vi "Impedance tube v1.0.1.vi"() -> ()   [LabVIEW 2021]
uses:
  <vilib>/Analysis/1siggen.llb/Ramp Pattern by Samples.vi
  <vilib>/express/express analysis/Spectral/Block/exnSpectralBlock spectral measurements RMS poly.vi
  <vilib>/express/express analysis/Spectral/Block/exnSpectralBlock spectral measurements RMS DDT.vi
  <vilib>/express/express arith-compare/Formula/XNode/ExpressFormulaBlockNode.xnode
  <vilib>/express/express analysis/Spectral/XNode/ExpressSpectralMeasurementsBlockNode.xnode
  <vilib>/Analysis/NI_AALPro.lvlib
  <vilib>/Analysis/NI_AALBase.lvlib
panel:
  out "Probe":dbl[](graph)
  out "Rr":dbl[](graph)
  out "Absorption coeff":dbl[](graph)
  in  "number of samples":i32=2048
  out "MIC 2":dynamicdata(graph)
  out "MIC 2":dbl
  out "FFT1":dynamicdata(graph)
  out "MIC 1":dynamicdata(graph)
  out "MIC 1":dbl
  in  "stop (F)":bool
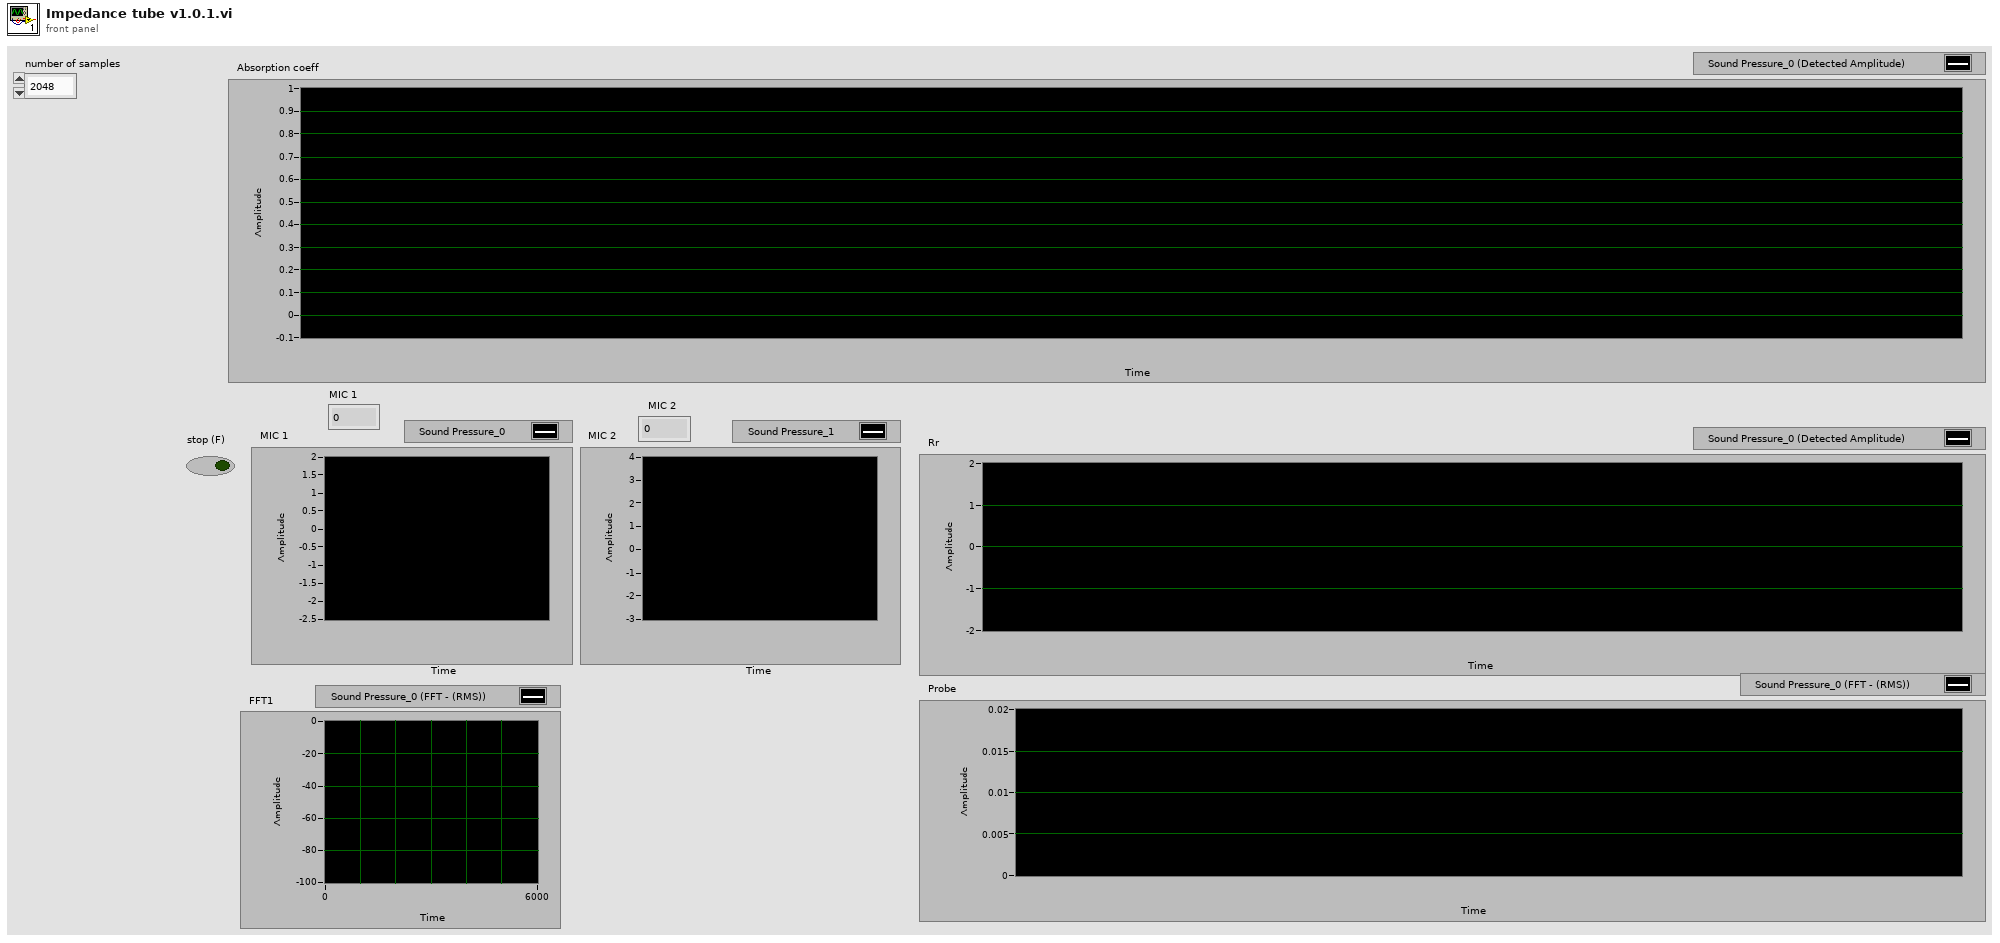
[diagram p1: front panel]
types:
  T1 = cluster{"averaging mode":u16, "weighting mode":u16, "number of averages":u32}
  T2 = cluster{"dB On (F)":bool, "unwrap phase (F)":bool, "convert to degree (F)":bool}
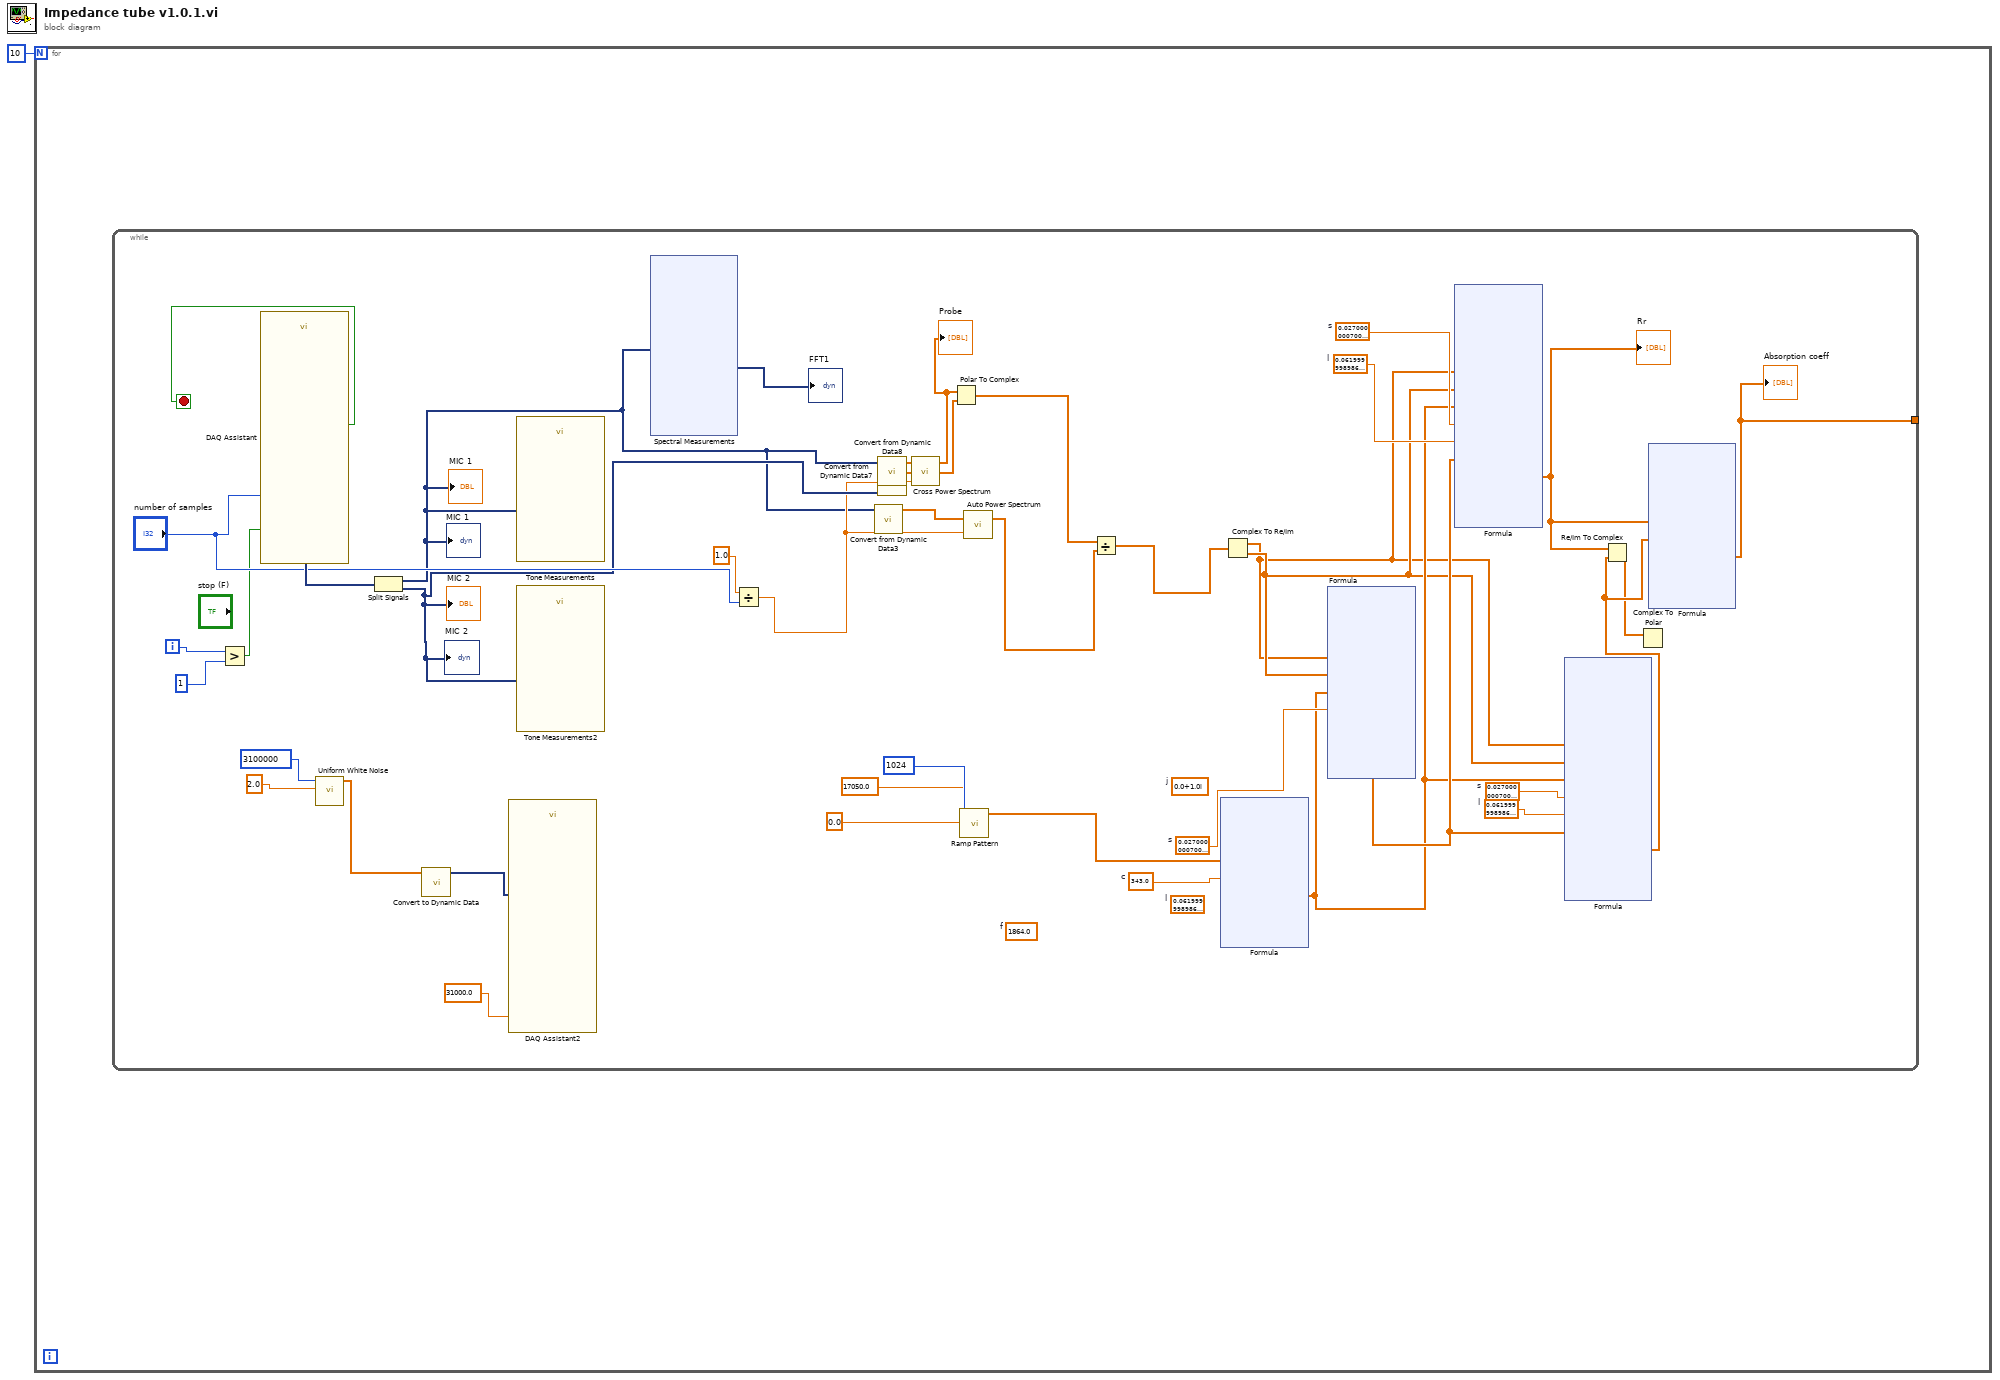
[diagram p0: block diagram]
diagram:
  n1 = for {
    N: 10 -> [_]
    n2 = while {
      tunnel: [w7] -> _
      i -> [w32]
      stop <- w8 stop-if-true
      w37 = sgl 0.062  # l
      w38 = sgl 0.027  # s
      w39 = sgl 0.062  # l
      w40 = sgl 0.027  # s
      (unwired) sgl 0.062  # l
      (unwired) sgl 1864.0  # f
      w41 = sgl 0.027  # s
      w42 = sgl 343.0  # c
      (unwired) csg 0.0+1.0i  # j
      n3 = Greater?(x=w32, y=1) -> (0:w9:bool)
      n4 = call "DAQ Assistant"("number of samples"="number of samples", "stop (F)"=w9) -> ("data"=w43:dynamicdata, "stopped"=w8:bool)  [unwired: 14 in, 2 out]
      n5 = call <vilib>:"Uniform White Noise.vi"("amplitude"=2.0, "samples"=3100000) -> ("uniform white noise"=w5:dbl[])  [unwired: 8 in, 1 out]
      n6 = Split Signals(w43) -> (w18:dynamicdata, w23:dynamicdata)  [unwired: 2 in]
      "MIC 1" <- w18
      "MIC 1" <- w18
      "MIC 2" <- w23
      "MIC 2" <- w23
      n7 = call "Convert to Dynamic Data"("Array"=w5) -> ("Dynamic Data Type"=w6:dynamicdata)  [unwired: 3 in]
      n8 = call "DAQ Assistant2"("data"=w6, "rate"=31000.0) -> ()  [unwired: 16 in, 2 out]
      n9 = call "Tone Measurements"("Signals"=w18) -> ()  [unwired: 8 in, 3 out]
      n10 = call "Tone Measurements2"("Signals"=w23) -> ()  [unwired: 8 in, 3 out]
      n11 = xnode "Spectral Measurements"("Signals"=w18) -> ("FFT - (RMS)"=→"FFT1":dynamicdata)  [unwired: 1 in, 2 out]
      n12 = Divide(x=1.0, y="number of samples") -> (x/y=w20:dbl)
      n13 = call "Convert from Dynamic Data3"("Dynamic Data Type"=w18) -> ("Array"=w17:dbl[])  [unwired: 3 in]
      n14 = call "Convert from Dynamic Data7"("Dynamic Data Type"=w18) -> ("Array"=w24:dbl[])  [unwired: 3 in]
      n15 = call "Convert from Dynamic Data8"("Dynamic Data Type"=w23) -> ("Array"=w22:dbl[])  [unwired: 3 in]
      n16 = call <vilib>:"Cross Power Spectrum.vi"("dt"=w20, "Signal Y (V)"=w22, "Signal X (V)"=w24) -> ("Cross Power XY Spectrum Phase (radians)"=w21:dbl[], "Cross Power XY Spectrum Mag (V^2rms)"=w19:dbl[])  [unwired: 1 out]
      "Probe" <- w19
      n17 = Polar To Complex(1:w21, 2:w19) -> (0:w16:cdb[])
      n18 = call-poly <vilib>:"Ramp Pattern.vi"("start"=0.0, "end"=17050.0, "samples"=1024) -> ("Ramp Pattern"=w10:dbl[])  [unwired: 7 in, 1 out]
      n19 = call <vilib>:"Auto Power Spectrum.vi"("dt"=w20, "Signal (V)"=w17) -> ("Power Spectrum (V^2 rms)"=w15:dbl[])  [unwired: 1 out]
      n20 = Divide(x=w16, y=w15) -> (x/y=w14:cdb[])
      n21 = xnode "Formula"("f"=w10, "c"=w42) -> ("Result"=w35:dbl[])  [unwired: 1 in, 1 out]
      n22 = Complex To Re/Im(x + iy=w14) -> (x=w29:dbl[], y=w34:dbl[])
      n23 = xnode "Formula"("Hr"=w29, "Hi"=w34, "k"=w35, "s"=w41) -> ("Result"=w36:dbl[])  [unwired: 1 in, 1 out]
      n24 = xnode "Formula"("Hr"=w29, "Hi"=w34, "k"=w35, "s"=w40, "l"=w39, "D"=w36) -> ("Result"=w26:dbl[])  [unwired: 1 in, 1 out]
      "Rr" <- w26
      n25 = xnode "Formula"("Hr"=w29, "Hi"=w34, "k"=w35, "s"=w38, "l"=w37, "D"=w36) -> ("Result"=w33:dbl[])  [unwired: 1 in, 1 out]
      n26 = Re/Im To Complex(1:w33, 2:w26) -> (0:w30:cdb[])
      n27 = Complex To Polar(r * e^(i*theta)=w30) -> ()  [unwired: 2 out]
      n28 = xnode "Formula"("Rr"=w26, "Ri"=w33) -> ("Result"=w7:dbl[])  [unwired: 1 in, 1 out]
      "Absorption coeff" <- w7
    }
  }
